vi "GoTo.vi"(3 "错误输入（无错误）":errorcluster, 5 "名称或相对路径":path) -> (0 "错误输出":errorcluster)   [LabVIEW 2023]
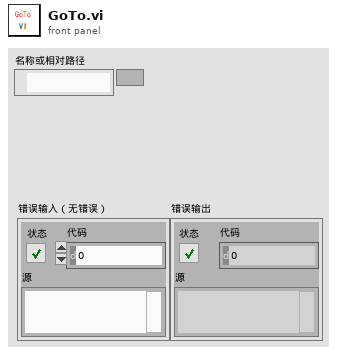
[diagram p1: front panel]
types:
  T1 = enum32{"Invalid", "Standard", "Closed", "Hidden", "Minimized", "Maximized"}
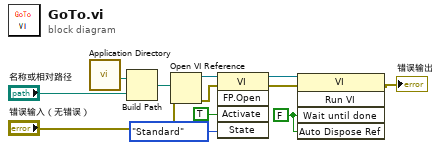
[diagram p0: block diagram]
diagram:
  w6 = FALSE ("结束前等待")
  n1 = call <vilib>:"Application Directory.vi"() -> ("Application Directory"=w7:path)
  n2 = Build Path(base path=w7, name or relative path="名称或相对路径") -> (appended path=w12:path)
  n3 = Open VI Reference(vi path=w12, error in (no error)="错误输入（无错误）") -> (vi reference=w11:refnum<vi>, error out=w10:errorcluster)  [unwired: 4 in]
  n4 = invoke class="VI" method="FP.Open"(reference=w11, error in=w10, "Activate"=TRUE ("激活？"), "State"=T1."Standard" ("状态")) -> (reference out=w9:refnum<vi>, error out=w8:errorcluster)  [unwired: 1 in, 3 out]
  n5 = invoke class="VI" method="Run VI"(reference=w9, error in=w8, "Wait until done"=w6, "Auto Dispose Ref"=w6) -> (error out=→"错误输出":errorcluster)  [unwired: 1 in, 4 out]
